vi "Configure Named Pattern.vi"(8 "error in (no error)":errorcluster, 9 "Operation (0: Active Existing Pattern)":i32(ring) items=["Active Existing Pattern", "Store Pattern", "Delete Pattern"], 10 "Pattern Name (PRBS_7)":string, 11 "VISA resource name":refnum<visa-resource-name>) -> (0 "error out":errorcluster, 3 "VISA resource name out":refnum<visa-resource-name>)   [LabVIEW 2009, in "Agilent 81150.lvlib"]
doc: "Configures the named pattern."
uses:
  Agilent 81150.lvlib
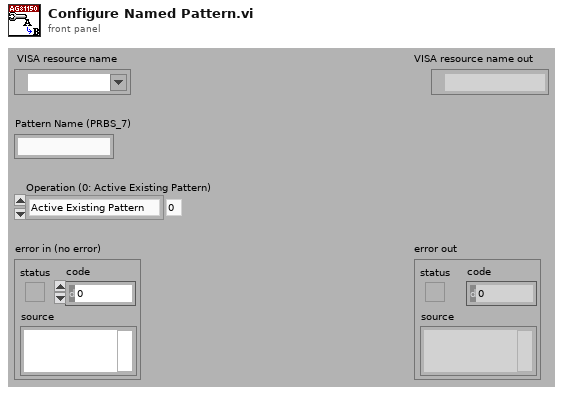
[diagram p1: front panel]
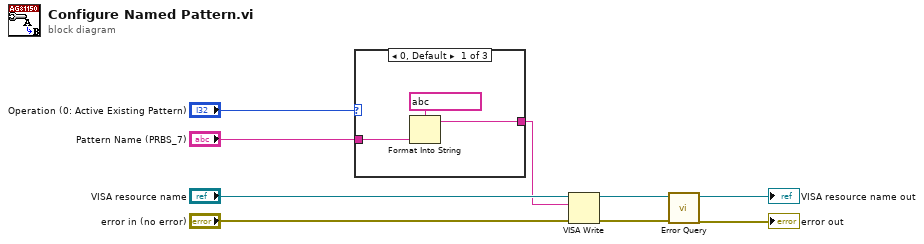
[diagram p0: block diagram]
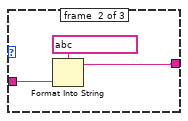
[diagram p2: hidden frame]
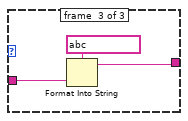
[diagram p3: hidden frame]
diagram:
  n1 = case shown="0, Default" "Operation (0: Active Existing Pattern)" {
    tunnel: "Pattern Name (PRBS_7)" -> [w11 w14 w17]
    tunnel: [w10 w13 w16] -> w1
    frame #0 {
      n2 = Format Into String(format string=string ?, w11) -> (resulting string=w10:string)  [unwired: 2 in, 1 out]
    }
    frame #1 {
      n3 = Format Into String(format string=string ?, w14) -> (resulting string=w13:string)  [unwired: 2 in, 1 out]
    }
    frame #2 {
      n4 = Format Into String(format string=string ?, w17) -> (resulting string=w16:string)  [unwired: 2 in, 1 out]
    }
  }
  n5 = VISA Write(VISA resource name="VISA resource name", write buffer=w1, error in (no error)="error in (no error)") -> (VISA resource name out=w7:refnum<visa-resource-name>, error out=w6:errorcluster)  [unwired: 1 out]
  n6 = call "Error Query.vi"("error in (no error)"=w6, "VISA resource name"=w7) -> ("error out"=→"error out":errorcluster, "VISA resource name out"=→"VISA resource name out":refnum<visa-resource-name>)  [unwired: 6 in, 2 out]
